vi "Write Athlete Profile Map.vi"(8 "error in (no error)":errorcluster, 10 "Athlete Profile Map":map{T1, T2}(c390), 11 "Data Manager in":refnum<class "Data Manager.lvclass">) -> (0 "error out":errorcluster, 3 "Data Manager out":refnum<class "Data Manager.lvclass">)   [LabVIEW 2020, in "Data Manager.lvclass"]
uses:
  Data Manager.lvclass
  Name--cluster.ctl
  Profile--cluster.ctl
  Data Manager.lvclass/Data Manager.ctl
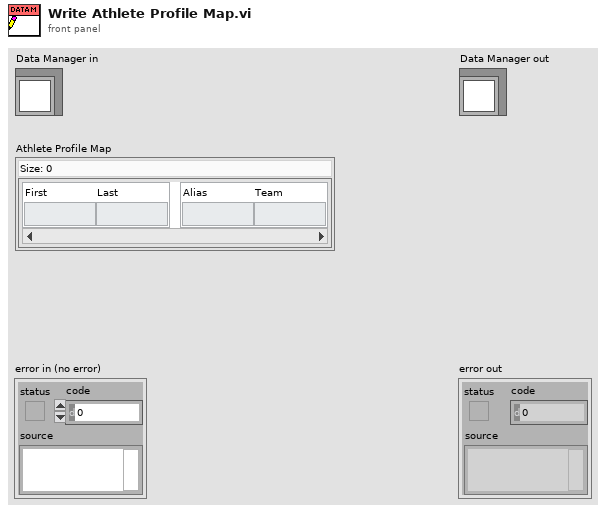
[diagram p1: front panel]
types:
  T1 = typedef "Data Manager.lvclass/Name--cluster.ctl" = cluster{"First":string, "Last":string}
  T2 = typedef "Data Manager.lvclass/Profile--cluster.ctl" = cluster{"Alias":string, "Team":string}
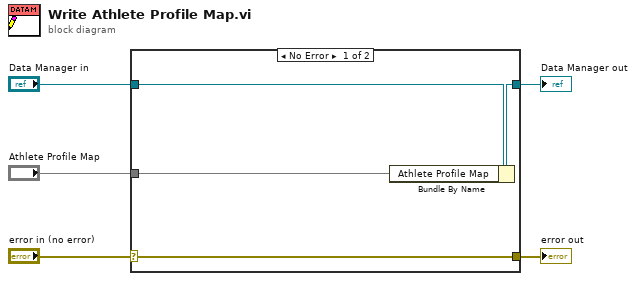
[diagram p0: block diagram]
diagram:
  n1 = case shown="No Error" "error in (no error)" {
    selector: "error in (no error)" -> [w9 w10]
    tunnel: [w9 w10] -> w4
    tunnel: [w7 w11] -> w2
    tunnel: "Data Manager in" -> [w8 w11]
    tunnel: "Athlete Profile Map" -> [w6 _]
    frame No Error {
      n2 = Bundle By Name(cluster=w8, "Athlete Profile Map"=w6) -> (w7:refnum<class "Data Manager.lvclass">)
    }
    frame Error {
    }
  }
  "error out" <- w4
  "Data Manager out" <- w2
